vi "MCP3422 Read 4 bytes.vi"(0 "VISA Refnum in":refnum<visa-resource-name>, 11 "error in (no error)":errorcluster) -> (4 "VISA Refnum out":refnum<visa-resource-name>, 6 "1st data byte":u8, 8 "2nd data byte":u8, 10 "3rd data byte":u8, 14 "configuration byte":u8, 15 "error out":errorcluster)   [LabVIEW 2015]
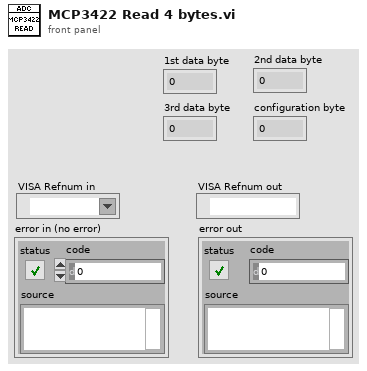
[diagram p1: front panel]
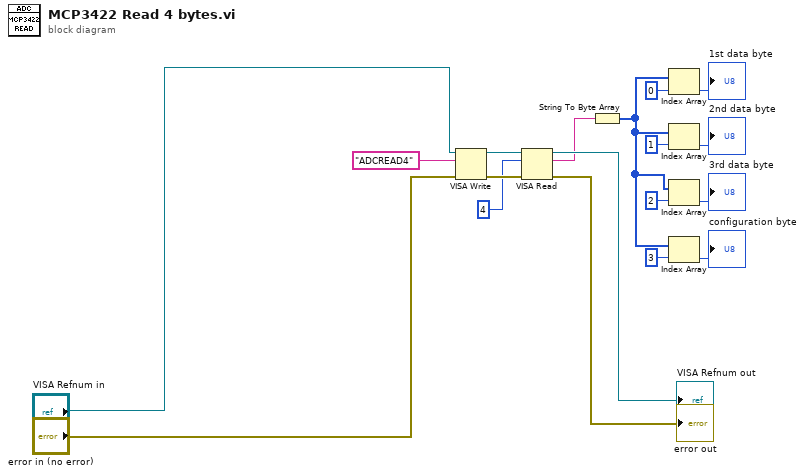
[diagram p0: block diagram]
diagram:
  n1 = VISA Write(VISA resource name="VISA Refnum in", write buffer="ADCREAD4", error in (no error)="error in (no error)") -> (VISA resource name out=w16:refnum<visa-resource-name>, error out=w15:errorcluster)  [unwired: 1 out]
  n2 = VISA Read(VISA resource name=w16, byte count=u32 4, error in (no error)=w15) -> (VISA resource name out=→"VISA Refnum out":refnum<visa-resource-name>, read buffer=w11:string, error out=→"error out":errorcluster)  [unwired: 1 out]
  n3 = String To Byte Array(string=w11) -> (unsigned byte array=w2:u8[])
  n4 = Index Array(array=w2, index=0) -> (element=→"1st data byte":u8)
  n5 = Index Array(array=w2, index=1) -> (element=→"2nd data byte":u8)
  n6 = Index Array(array=w2, index=2) -> (element=→"3rd data byte":u8)
  n7 = Index Array(array=w2, index=3) -> (element=→"configuration byte":u8)
